vi "Publish Audio Spectrum.vi"(8 "Error In":errorcluster, 10 "Audio Spectrum":dbl[](array[numeric]), 11 "Audio Analyzer In":refnum<class "Audio Analyzer.lvclass">) -> (0 "Error Out":errorcluster, 3 "Audio Analyzer Out":refnum<class "Audio Analyzer.lvclass">)   [LabVIEW 2021, in "Audio Analyzer.lvclass"]
uses:
  Audio Analyzer.lvclass
  Accessors/Audio Spectrum Notifier/Get Audio Spectrum Notifier.vi
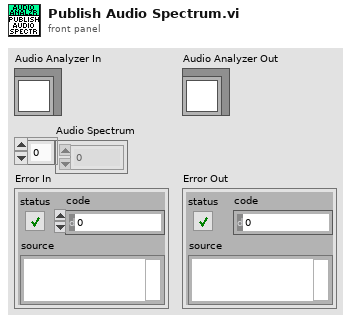
[diagram p1: front panel]
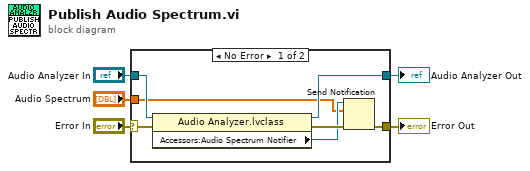
[diagram p0: block diagram]
diagram:
  n1 = case shown="No Error" "Error In" {
    selector: "Error In" -> [w12 w13]
    tunnel: [w6 w13] -> w5
    tunnel: "Audio Analyzer In" -> [w11 w14]
    tunnel: [w10 w14] -> w2
    tunnel: "Audio Spectrum" -> [w7 _]
    frame No Error {
      n2 = property class="Audio Analyzer.lvclass"(reference=w11, error in=w12) -> (reference out=w10:refnum<class "Audio Analyzer.lvclass">, error out=w9:errorcluster, "Accessors:Audio Spectrum Notifier"=w8:refnum<notifier>)
      n3 = Send Notification(notification=w7, notifier=w8, error in (no error)=w9) -> (error out=w6:errorcluster)  [unwired: 1 out]
    }
    frame Error {
    }
  }
  "Error Out" <- w5
  "Audio Analyzer Out" <- w2
